vi "Time Varying Filter.vi"() -> ()   [LabVIEW 2023]
doc: "This example shows how to use the TFA Time Varying Filter VI.\n\n<b>Instructions:</b>\n1) Run this VI to display the <b>Time Varying Filter</b> dialog box.\n2) Specify the filtering behavior in the dialog box.\n3) Click the <b>Accept</b> button to accept the filtering settings and to close the dialog box.\n4) Compare the original <b>Noisy signal</b> and <b>Denoised signal</b>."
uses:
  <vilib>/addons/Time Frequency Analysis/typedefs.llb/TFA Data.ctl
  <vilib>/addons/Time Frequency Analysis/Application.llb/TFA Time Varying Filter (Waveform).vi
  <vilib>/addons/_Advanced Signal Processing/NI_AdvSigProcTFA.lvlib
panel:
  out "aspt-left-top":bool
  out "Denoised Signal":waveform(dbl)(graph)
  out "Noisy Signal":waveform(dbl)(graph)
  # "Overview: Shows how to use the TFA Time Varying Filter VI.\nRequirements: LabVIEW Full Development System, Advanced Signal Processing Toolkit\nInstructions: \n1. Run this VI to display the Time Varying Filter dialog box.\n2. Specify the filtering behavior in the dialog box.\n3. Click the Accept button to accept the filtering settings and to close the dialog box.\n4. Compare the original Noisy signal and Denoised signal."
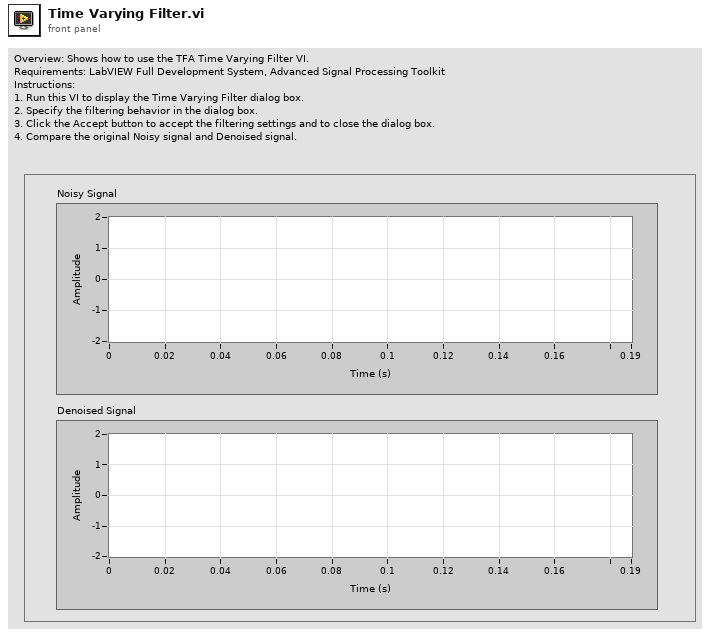
[diagram p1: front panel]
types:
  T1 = typedef "NI_AdvSigProcTFA.lvlib/TFA Data.ctl" = u16
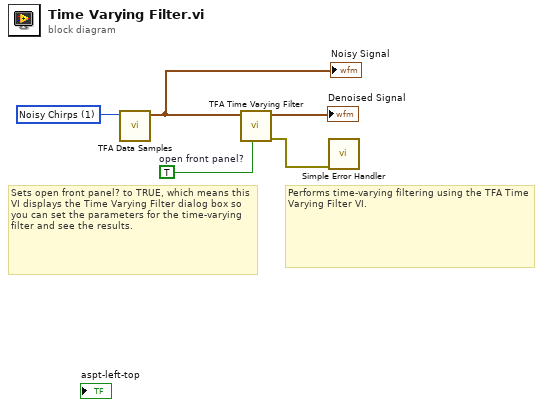
[diagram p0: block diagram]
diagram:
  w1 = TRUE  # open front panel?
  w3 = T1 1 items=["PC Fan"=0, "Noisy Chirps"=1, "TDR 1"=2, "TDR 2"=3, "Liquefaction"=4, "Liquefaction Free"=5, "Aneurysm"=6, "Bat"=7, "RF"=8, "Two Gaussian"=9, "Three Gaussian"=10, "Chirp"=11, "Gaussian Chirp"=12, "Cross Chirp"=13, "Doppler"=14, "HOP"=15, "TF Sine"=16, "Three Tone"=17, "Four Tone"=23, "Blood Flow Doppler (phase a)"=20, "Blood Flow Doppler (phase b)"=21, "Heart sound"=22, "-"=18, "Random Noise"=19] ("data")
  # "Sets open front panel? to TRUE, which means this VI displays the Time Varying Filter dialog box so you can set the parameters for the time-varying filter and see the results."
  # "Performs time-varying filtering using the TFA Time Varying Filter VI."
  n1 = call <vilib>:"TFA Data Samples.vi"("data"=w3) -> ("signal"=w5:waveform(dbl))  [unwired: 10 out]
  "Noisy Signal" <- w5
  n2 = call-poly <vilib>:"TFA Time Varying Filter.vi"("open front panel? (T)"=w1, "signal"=w5) -> ("error out"=w2:errorcluster, "filtered signal"=→"Denoised Signal":waveform(dbl))  [unwired: 2 in, 6 out]
  n3 = call <vilib>:"Simple Error Handler.vi"("error in (no error)"=w2) -> ()  [unwired: 4 in, 5 out]
